vi "AddRequest.vi"(5 "Reply Params Source":refnum<vi>, 7 "Request Params Source":refnum<vi>, 9 "Request Name":string, 10 "Module Name":string="TemplateModule", 11 "Module Ref":refnum<vi>) -> ()   [LabVIEW 2024, in "AddNewEvent.lvlib"]
uses:
  Event/AddNewEvent.lvlib
  <vilib>/Utility/miscctls.llb/LVPositionTypeDef.ctl
  <vilib>/_script/New VI Object TypeDefs/NewVIObject_LVRelativePositionTypeDef.ctl
  <vilib>/_script/New VI Object TypeDefs/NewVIObject_LVRelativeDirectionTypeDef.ctl
  <vilib>/Utility/miscctls.llb/LVPoint32TypeDef.ctl
  <vilib>/event_ctls.llb/lveventtype.ctl
  <vilib>/Utility/traverseref.llb/TRef TravTarget.ctl
  <vilib>/Utility/miscctls.llb/LVPointTypeDef.ctl
  templates/RequestTemplate.vi
  Event/Templates/EHLRequest.vi
  Event/Templates/RequestMessageTemplate.ctl
  <vilib>/addons/analyzer/_analyzerutils.llb/VIAnUtil Check Type If ErrClust.vi
  <vilib>/Utility/traverseref.llb/VI Scripting - Traverse.lvlib
  templates/TemplateModule/TemplateModule.Start.vi
  templates/TemplateModule/TemplateModule.lvclass
  <vilib>/Utility/Data Type/NI_Data Type.lvlib
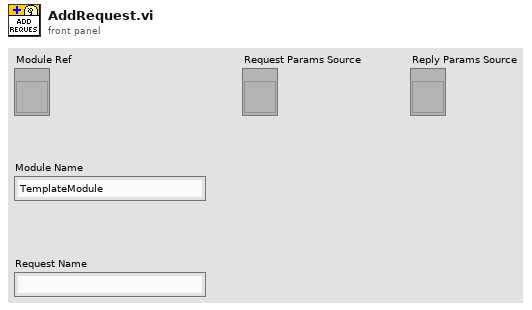
[diagram p1: front panel]
types:
  T1 = typedef "LVPositionTypeDef.ctl" = cluster{"Left":i32, "Top":i32}
  T2 = typedef "lveventtype.ctl" = enum32{"Null", "Timeout", "Annotation Menu Selection", "Annotation Menu Selection?", "App Instance Close", "App Instance Close?", "Autoscale Range Change", "Bookmark Info Change", "Cell Edit", "Cell Edit?", "Cursor Grab", "Cursor Grab?", "Cursor Menu Selection", "Cursor Menu Selection?", "Cursor Move", "Cursor Release", "Data Change", "Direction Change", "Display State Change", "Drag Ended", "Drag Enter", "Drag Leave", "Drag Over", "Drag Source Update", "Drag Starting", "Drag Starting?", "Drop", "Exec State Change", "Key Down", "Key Down?", "Key Repeat", "Key Repeat?", "Key Up", "Listbox Double Click", "Menu Activation?", "Menu Selection (App)", "Menu Selection? (App)", "Menu Selection (User)", "Mouse Down", "Mouse Down?", "Mouse Enter", "Mouse Leave", "Mouse Move", "Mouse Up", "Mouse Wheel", "NI Security User Change (App)", "Pane Size", "Panel Close", "Panel Close?", "Panel Resize", "Plot Attribute Change", "Scale Range Change", "Shortcut Menu Activation?", "Shortcut Menu Selection (App)", "Shortcut Menu Selection? (App)", "Shortcut Menu Selection (User)", "Tree Double Click", "Tree Drag", "Tree Drag?", "Tree Drop", "Tree Drop?", "Tree Item Close", "Tree Item Close?", "Tree Item Open", "Tree Item Open?", "User Event", "Value Change"}
  T3 = cluster{"Event Type":T2, "Reference":refnum<vi>, "Limit (-1=none)":i32, "Lock Panel?":bool}
  T4 = typedef "LVPointTypeDef.ctl" = cluster{"Horizontal":i16, "Vertical":i16}
  T5 = typedef "TRef TravTarget.ctl" = enum16{"FP", "BD", "Other"}
  T6 = enum32{"invalid VI type", "Standard VI", "Control VI", "Global VI", "Polymorphic VI", "Configuration VI", "SubSystem", "Facade VI", "Method VI", "Statechart Diagram VI"}
  T7 = cluster{"Event Type":T2, "Event Registration Index":i32}
  T8 = typedef "NewVIObject_LVRelativePositionTypeDef.ctl" = cluster{"Refnum":refnum<vi>, "Relative Direction":T9, "Point32":T10}
  T9 = typedef "NewVIObject_LVRelativeDirectionTypeDef.ctl" = enum32{"Right", "Left", "Top", "Bottom", "Top Right", "Top Left", "Bottom Right", "Bottom Left"}
  T10 = typedef "LVPoint32TypeDef.ctl" = cluster{"Horizontal":i32, "Vertical":i32}
  T11 = cluster{"Event Type":T2, "Event Registration Index":i32}[]
  T12 = cluster{"Event Type":T2, "Reference":refnum<vi>, "Limit (-1=none)":i32, "Lock Panel?":bool}[]
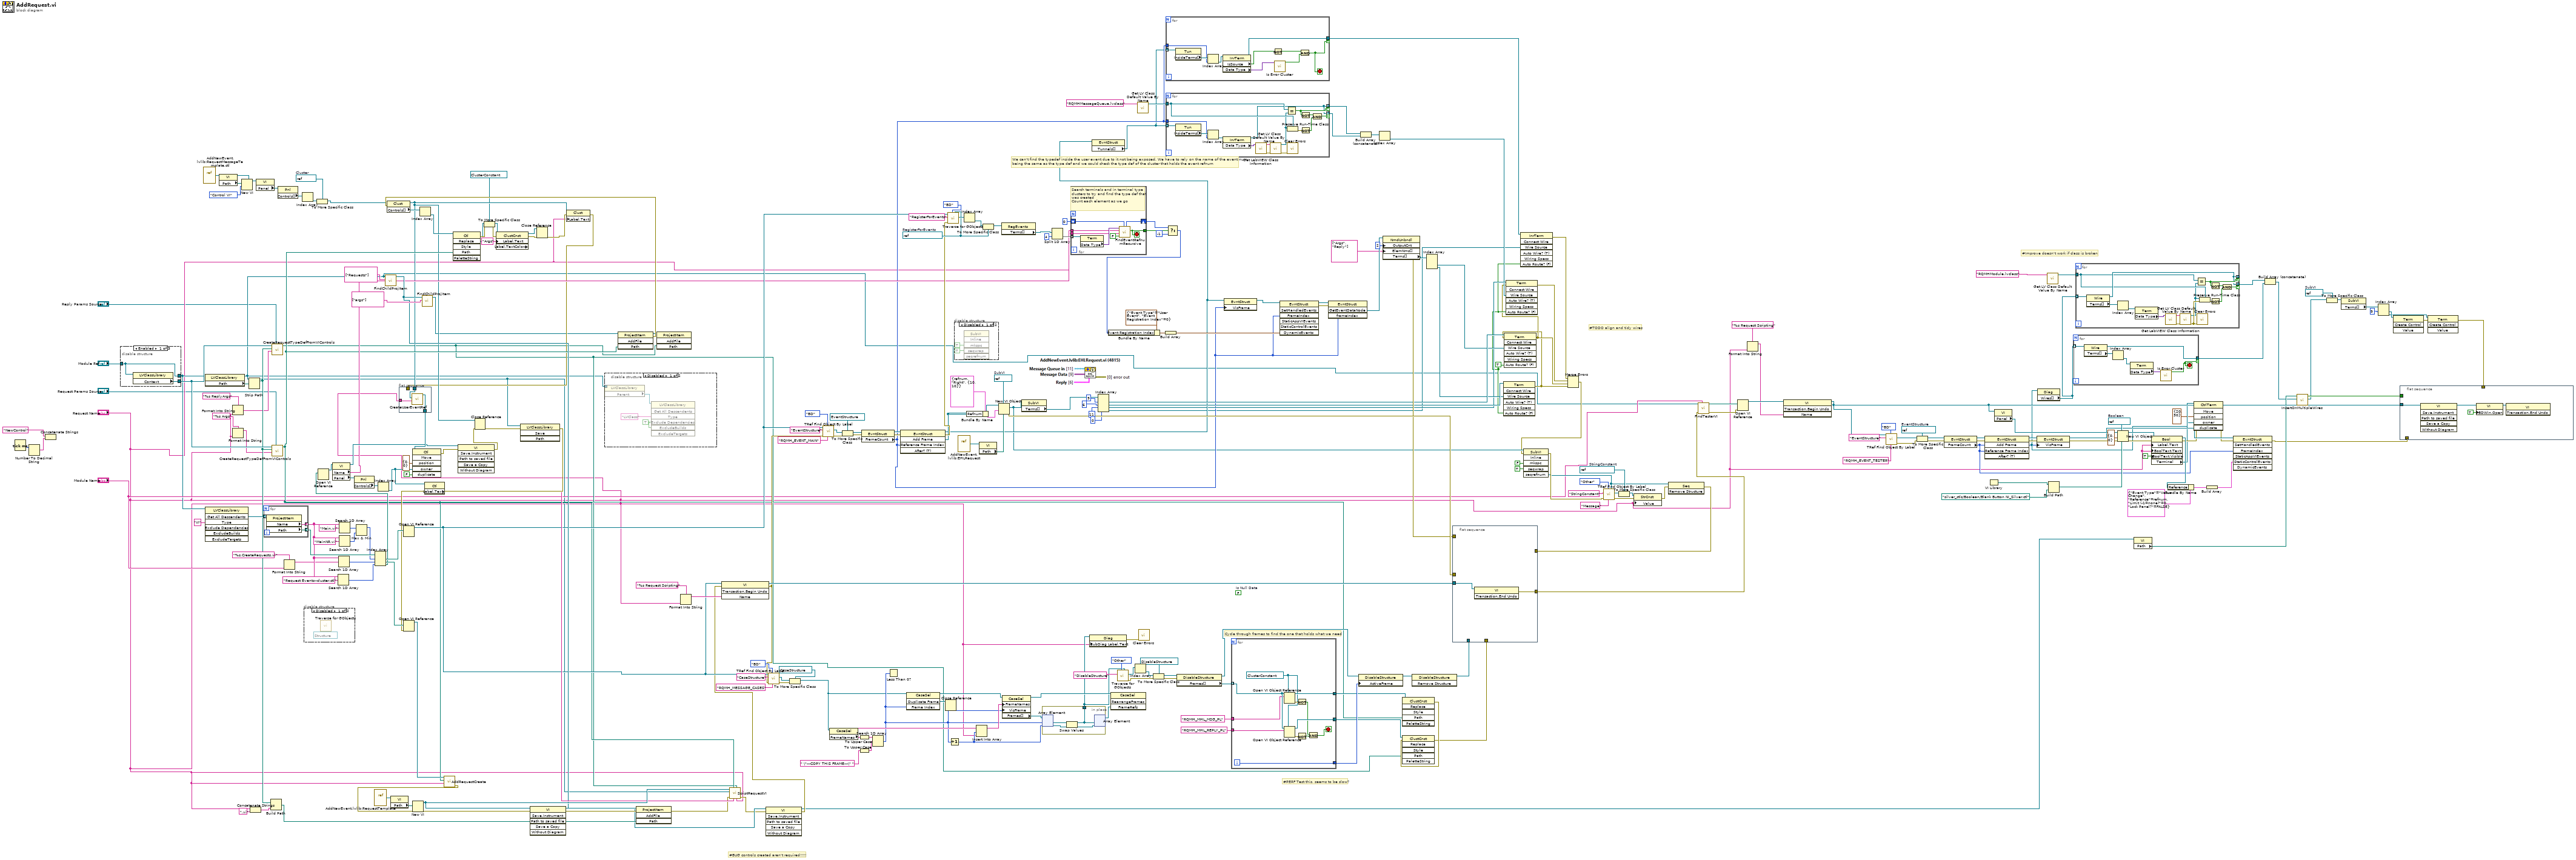
[diagram p0: block diagram]
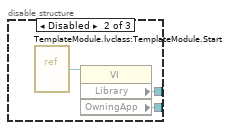
[diagram p2: hidden frame]
diagram:
  w12 = refnum<vi> refnum  # SubVI
  w40 = refnum<vi> refnum  # Boolean
  w58 = refnum<vi> refnum  # EventStructure
  w82 = refnum<vi> refnum  # StringConstant
  w93 = TRUE ("Auto Route? (F)")
  w139 = refnum<vi> refnum  # Cluster
  w170 = refnum<vi> refnum  # RegisterForEvents
  w200 = refnum<vi> refnum  # SubVI
  (unwired) FALSE  # Is Null Data
  # "#BUG controls created aren't required!!!!!"
  # "#Improve doesn't work if class is broken"
  # "#TODO align and tidy wires"
  # "We can't find the typedef inside the user event due to it not being exposed. We have to rely on the name of the event num\nbeing the same as the type def and we could check the type def of the cluster that holds the event refnum"
  # "#PERF Test this, seems to be slow?"
  # "Cycle through frames to find the one that holds what we need"
  n1 = Tick Count (ms)() -> (millisecond timer value=w278:u32)
  n2 = Number To Decimal String(number=w278) -> (decimal integer string=w277:string)  [unwired: 1 in]
  n3 = Concatenate Strings("NewControl", w277) -> ()  [unwired: 1 out]
  n4 = disable-structure shown="Enabled" {
    disable-tunnel: [w282 w285 _] -> w17
    disable-tunnel: [w283 w284 _] -> w213
    disable-tunnel: "Module Ref" -> [w282 _ _]
    frame Enabled {
      n5 = property class="LVClassLibrary"(reference=w282) -> ("Context"=w283:refnum<vi>)  [unwired: 1 in, 2 out]
    }
    frame Disabled {
      n6 = vi-ref "TemplateModule.lvclass:TemplateModule.Start.vi"() -> (w286:refnum<vi>)
      n7 = property class="VI"(reference=w286) -> ("Library"=w285:refnum<vi>, "OwningApp"=w284:refnum<vi>)  [unwired: 1 in, 2 out]
    }
    frame Disabled {
    }
  }
  n8 = vi-ref "AddNewEvent.lvlib:RequestMessageTemplate.ctl"() -> (w147:refnum<vi>)
  n9 = property class="LVClassLibrary"(reference=w17) -> (reference out=w68:refnum<vi>, "Path"=w281:path)  [unwired: 1 in, 1 out]
  n10 = invoke class="LVClassLibrary" method="Get All Descendents"(reference=w17, "Type"="VI") -> ("All Descendents"=w274:refnum<vi>[])  [unwired: 5 in, 6 out]
  n11 = property class="VI"(reference=w147) -> (reference out=w140:refnum<vi>, "Path"=w146:path)  [unwired: 1 in, 1 out]
  n12 = Format Into String(format string="%s ReplyArgs", "Request Name") -> (resulting string=w211:string)  [unwired: 2 in, 1 out]
  n13 = Format Into String(format string="%s Args", "Request Name") -> (resulting string=w208:string)  [unwired: 2 in, 1 out]
  n14 = New VI(5:w140, 9:T6."Control VI" ("vi type (standard vi)"), 10:w146) -> (3:w142:refnum<vi>)  [unwired: 4 in, 1 out]
  n15 = Strip Path(path=w281) -> (stripped path=w212:path)  [unwired: 1 out]
  n16 = Concatenate Strings("Request Name", ".vi" ("string")) -> (w248:string)
  n17 = property class="VI"(reference=w142) -> ("Panel"=w144:refnum<vi>)  [unwired: 1 in, 2 out]
  n18 = for {
    tunnel: w274 -> [w289] mode=indexing
    tunnel: [w288] -> w260 mode=indexing
    tunnel: [w287] -> w269 mode=indexing
    n19 = property class="ProjectItem"(reference=w289) -> ("Name"=w288:string, "Path"=w287:path)  [unwired: 1 in, 2 out]
  }
  n20 = Build Path(base path=w212, name or relative path=w248) -> (appended path=w247:path)
  n21 = call "CreateRequestTypeDefFromVIControls.vi"("VI Refnum"="Reply Params Source", "Control Name"=w211, "SaveFolderPath"=w212, "Application in"=w213) -> ("TypeDef Path"=w70:path)  [unwired: 6 in, 1 out]
  n22 = call "CreateRequestTypeDefFromVIControls.vi"("VI Refnum"="Request Params Source", "Control Name"=w208, "SaveFolderPath"=w212, "Application in"=w213) -> ("TypeDef Path"=w135:path)  [unwired: 6 in, 1 out]
  n23 = property class="Pnl"(reference=w144) -> ("Controls[]"=w143:refnum<vi>[])  [unwired: 1 in, 2 out]
  n24 = Format Into String(format string="%s.CreateRequests.vi" ("element"), "Module Name") -> (resulting string=w239:string)  [unwired: 2 in, 1 out]
  n25 = Index Array(array=w143) -> (element=w141:refnum<vi>)  [unwired: 1 in]
  n26 = disable-structure shown="Disabled" {
    frame Disabled {
      (unwired) refnum<vi> refnum ("Struct Refnum")
      n27 = call <vilib>:"Traverse for GObjects.vi"() -> ()  [unwired: 8 in, 4 out]
    }
    frame Enabled {
    }
  }
  n28 = To More Specific Class(target class=w139, reference=w141) -> (specific class reference=w138:refnum<vi>)  [unwired: 1 in, 1 out]
  n29 = Search 1D Array(1D array=w260, element="Request Events--cluster.ctl") -> (index of element=w259:i32)  [unwired: 1 in]
  n30 = Search 1D Array(1D array=w260, element=w239) -> (index of element=w268:i32)  [unwired: 1 in]
  n31 = Search 1D Array(1D array=w260, element="Main.vi") -> (index of element=w271:i32)  [unwired: 1 in]
  n32 = Search 1D Array(1D array=w260, element="MainNR.vi") -> (index of element=w270:i32)  [unwired: 1 in]
  n33 = Max & Min(x=w271, y=w270) -> (max(x,y)=w267:i32)  [unwired: 1 out]
  n34 = vi-ref "AddNewEvent.lvlib:RequestTemplate.vi"() -> (w280:refnum<vi>)
  n35 = Index Array(array=w269, index #1=w267, index #2=w268, index #3=w259) -> (element #1=w265:path, element #2=w266:path, element #3=w255:path)
  n36 = Open VI Reference(vi path=w255) -> (vi reference=w256:refnum<vi>)  [unwired: 5 in, 1 out]
  n37 = property class="VI"(reference=w256) -> (reference out=w205:refnum<vi>, "Name"=w157:string, "Panel"=w258:refnum<vi>)  [unwired: 1 in, 1 out]
  n38 = property class="Pnl"(reference=w258) -> ("Controls[]"=w257:refnum<vi>[])  [unwired: 1 in, 2 out]
  n39 = Index Array(array=w257) -> (element=w245:refnum<vi>)  [unwired: 1 in]
  n40 = call "FindChildProjItem.vi"("Level"=string[] ["Requests"], "ProjectItem in"=w68) -> ("Found or Orig"=w201:refnum<vi>)  [unwired: 8 in, 1 out]
  n41 = property class="VI"(reference=w280) -> ("Path"=w279:path)  [unwired: 1 in, 2 out]
  n42 = flat-sequence {
    tunnel: [w292] -> w252
    tunnel: "Request Name" -> [w291]
    tunnel: w131 -> [w290]
    tunnel: w129 -> [_]
    frame #0 {
      n43 = call "CreateUserEventRef.vi"("Label.Text"=w291, "referenceToEventRef"=w290) -> ("UserEventCtlRef"=w292:refnum<vi>)  [unwired: 9 in]
    }
  }
  n44 = Open VI Reference(vi path=w265) -> (vi reference=w160:refnum<vi>)  [unwired: 5 in, 1 out]
  n45 = invoke class="Ctl" method="Move"(reference=w252, "position"=T1 {"Left"=0, "Top"=0}, "owner"=w245, "duplicate"=FALSE ("Duplicate? (F)")) -> (error out=w207:errorcluster)  [unwired: 2 in, 5 out]
  n46 = call "FindChildProjItem.vi"("Level"=string[] ["args"], "ProjectItem in"=w201) -> ("Found or Orig"=w120:refnum<vi>)  [unwired: 8 in, 1 out]
  n47 = property class="Ctl"(reference=w245) -> ("Label.Text"=w244:string)  [unwired: 1 in, 2 out]
  n48 = invoke class="VI" method="Save.Instrument"(reference=w205, error in=w207) -> (error out=w206:errorcluster)  [unwired: 4 in, 5 out]
  n49 = disable-structure shown="Disabled" {
    disable-tunnel: w68 -> [w296 _]
    frame Disabled {
      w294 = TRUE ("ExcludeDependencies")
      n50 = property class="LVClassLibrary"(reference=w296) -> ("Parent"=w295:refnum<vi>)  [unwired: 1 in, 2 out]
      n51 = invoke class="LVClassLibrary" method="Get All Descendents"(reference=w295, "Type"="LVClass", "Exclude Dependencies"=w294, "ExcludeBuilds"=w294) -> ()  [unwired: 3 in, 7 out]
    }
    frame Enabled {
    }
  }
  n52 = invoke class="ProjectItem" method="AddFile"(reference=w120, "Path"=w135) -> (reference out=w121:refnum<vi>, error out=w204:errorcluster)  [unwired: 2 in, 2 out]
  n53 = property class="Clust"(reference=w138, error in=w204) -> (reference out=w131:refnum<vi>, "Controls[]"=w137:refnum<vi>[])  [unwired: 1 out]
  n54 = Index Array(array=w137) -> (element=w136:refnum<vi>)  [unwired: 1 in]
  n55 = invoke class="Ctl" method="Replace"(reference=w136, "Path"=w135) -> (error out=w128:errorcluster, "Replace"=w126:refnum<vi>)  [unwired: 4 in, 4 out]
  n56 = Close Reference(reference=w131, error in (no error)=w206) -> (error out=w263:errorcluster)
  n57 = To More Specific Class(target class=refnum<vi> refnum ("ClustCnst Refnum"), reference=w126, error in=w128) -> (specific class reference=w124:refnum<vi>, error out=w127:errorcluster)
  n58 = property class="ClustCnst" props=["Label", "Text", "Label", "TextColors"](reference=w124, error in=w127, "Label.Text"="Args") -> (reference out=w133:refnum<vi>, error out=w132:errorcluster)  [unwired: 1 out]
  n59 = invoke class="LVClassLibrary" method="Save"(reference=w68, error in=w263) -> (error out=w254:errorcluster)  [unwired: 2 in, 3 out]
  n60 = Open VI Reference(vi path=w266, error in (no error)=w254) -> (vi reference=w264:refnum<vi>)  [unwired: 4 in, 1 out]
  n61 = call "AddRequestCreate.vi"("New Name"="Request Name", "TypeDefPath"=w135, "VI in"=w264) -> ("error out"=w149:errorcluster)  [unwired: 8 in]
  n62 = New VI(8:w149, 10:w279) -> (0:w251:errorcluster, 3:w246:refnum<vi>)  [unwired: 5 in]
  n63 = invoke class="VI" method="Save.Instrument"(reference=w246, error in=w251, "Path to saved file"=w247) -> (reference out=w48:refnum<vi>, error out=w250:errorcluster)  [unwired: 3 in, 4 out]
  n64 = Close Reference(reference=w133, error in (no error)=w132) -> (error out=w130:errorcluster)
  n65 = property class="Clust"(reference=w131, error in=w130, "Label.Text"="Request Name") -> (error out=w129:errorcluster)  [unwired: 1 out]
  n66 = invoke class="ProjectItem" method="AddFile"(reference=w201, error in=w250, "Path"=w247) -> (error out=w148:errorcluster)  [unwired: 1 in, 3 out]
  n67 = invoke class="ProjectItem" method="AddFile"(reference=w121, "Path"=w70) -> ()  [unwired: 2 in, 4 out]
  n68 = Format Into String(format string="%s Request Scripting", "Request Name") -> (resulting string=w178:string)  [unwired: 2 in, 1 out]
  n69 = call "ScriptRequestVI.vi"("Request Name"="Request Name", "REPLYTypeDef Path"=w70, "EventClusterName"=w244, "REQTypeDef Path"=w135, "error in (no error)"=w148, "Module Ref"=w68, "VI in"=w246) -> ("error out"=w47:errorcluster)  [unwired: 4 in]
  n70 = invoke class="VI" method="Save.Instrument"(reference=w48, error in=w47) -> (reference out=w45:refnum<vi>, error out=w46:errorcluster)  [unwired: 4 in, 4 out]
  n71 = invoke class="VI" method="Transaction.Begin Undo"(reference=w160, error in=w46, "Name"=w178) -> (reference out=w177:refnum<vi>, error out=w159:errorcluster)  [unwired: 1 in, 2 out]
  n72 = call <vilib>:"TRef Find Object By Label.vi"("Label"="RQMH_MESSAGE_CASES", "Traverse Target"=TRef_TravTarget."BD", "error in (no error)"=w159, "Class Name"="CaseStructure", "VI Ref"=w160) -> ("error out"=w181:errorcluster, "Found Obj Ref"=w182:refnum<vi>)  [unwired: 3 in, 2 out]
  n73 = To More Specific Class(target class=refnum<vi> refnum ("CaseSel Refnum"), reference=w182, error in=w181) -> (specific class reference=w180:refnum<vi>)  [unwired: 1 out]
  n74 = call <vilib>:"TRef Find Object By Label.vi"("Label"="RQMH_EVENT_MAIN", "Traverse Target"=TRef_TravTarget."BD", "error in (no error)"=w159, "Class Name"="EventStructure", "VI Ref"=w160) -> ("error out"=w196:errorcluster, "Found Obj Ref"=w195:refnum<vi>)  [unwired: 3 in, 2 out]
  n75 = property class="CaseSel"(reference=w180) -> ("FrameNames"=w225:string[])  [unwired: 1 in, 2 out]
  n76 = To More Specific Class(target class=refnum<vi> refnum ("EvntStruct Refnum"), reference=w195, error in=w196) -> (specific class reference=w191:refnum<vi>, error out=w193:errorcluster)
  n77 = To Upper Case(1:" \"---COPY THIS FRAME---\" " ("key")) -> (0:w237:string)
  n78 = To Upper Case(1:w225) -> (0:w238:string[])
  n79 = property class="EvntStruct"(reference=w191, error in=w193) -> (reference out=w174:refnum<vi>, error out=w192:errorcluster, "FrameCount"=w97:i32)
  n80 = Search 1D Array(1D array=w238, element=w237) -> (index of element=w222:i32)  [unwired: 1 in]
  n81 = Less Than 0?(x=w222) -> ()  [unwired: 1 out]
  n82 = invoke class="EvntStruct" method="Add Frame"(reference=w174, error in=w192, "Reference Frame Index"=w97) -> (reference out=w107:refnum<vi>, error out=w158:errorcluster, "Add Frame"=w108:refnum<vi>)  [unwired: 2 in, 2 out]
  n83 = invoke class="CaseSel" method="Duplicate Frame"(reference=w180, "Frame Index"=w222) -> (reference out=w235:refnum<vi>, "Duplicate Frame"=w231:refnum<vi>)  [unwired: 2 in, 2 out]
  n84 = Close Reference(reference=w231) -> ()  [unwired: 1 in, 1 out]
  n85 = call <vilib>:"Traverse for GObjects.vi"("Other Refnum"=w170, "Traverse Target"=TRef_TravTarget."BD", "error in (no error)"=w158, "Class Name"="RegisterForEvents", "VI Refnum"=w160) -> ("References"=w171:refnum<vi>[])  [unwired: 3 in, 3 out]
  n86 = Increment(x=w222) -> (x+1=w223:i32)
  n87 = disable-structure shown="Disabled" {
    frame Disabled {
      n88 = invoke class="SubVI" method="Inline"("mkspc"=TRUE ("Make Space in Block Diagram"), "seqwrap"=TRUE ("Wrap in Sequence")) -> ()  [unwired: 4 in, 6 out]
    }
    frame Enabled {
    }
  }
  n89 = vi-ref "AddNewEvent.lvlib:EHLRequest.vi"() -> (w189:refnum<vi>)
  n90 = Index Array(array=w171) -> (element=w169:refnum<vi>)  [unwired: 1 in]
  n91 = Bundle By Name(cluster=T8 {"Refnum"=refnum, "Relative Direction"=enum."Right", "Point32"={"Horizontal"=10, "Vertical"=10}} ("Relative Position"), "Refnum"=w108) -> (w187:T8)
  n92 = Insert Into Array(array=w225, index=w223, new element="Request Name") -> (w224:string[])
  n93 = property class="VI"(reference=w189) -> ("Path"=w188:path)  [unwired: 1 in, 2 out]
  n94 = To More Specific Class(target class=w170, reference=w169) -> (specific class reference=w168:refnum<vi>)  [unwired: 1 in, 1 out]
  n95 = New VI Object(vi object class=w200, owner refnum=w108, position/next to=w187, 6:w188) -> (object refnum=w89:refnum<vi>, 0:w175:errorcluster)  [unwired: 4 in]
  n96 = property class="RegEvents"(reference=w168) -> ("Terms[]"=w167:refnum<vi>[])  [unwired: 1 in, 2 out]
  n97 = property class="CaseSel"(reference=w235, "FrameNames"=w224, "VisFrame"=w222) -> (reference out=w234:refnum<vi>, "Frames[]"=w233:refnum<vi>[])  [unwired: 1 in, 1 out]
  n98 = property class="SubVI"(reference=w89) -> ("Terms[]"=w116:refnum<vi>[])  [unwired: 1 in, 2 out]
  n99 = in-place {
    in-place-border: [w299] -> w226
    n100 = in-place-array #1(w233, w222, w223) -> (w302:refnum<vi>, w301:refnum<vi>)
    n101 = Swap Values(12:w302, 14:w301) -> (1:w299:refnum<vi>, 3:w300:refnum<vi>)  [unwired: 1 in]
    n102 = in-place-array #1(w299, w300) -> (w232:refnum<vi>[])  [unwired: 2 out]
  }
  n103 = Split 1D Array(array=w167, index=4) -> (second subarray=w165:refnum<vi>[])  [unwired: 1 out]
  n104 = for {
    tunnel: w165 -> [w310] mode=indexing
    tunnel: "Request Name" -> [w305]
    shift-right: [w309] -> w161
    shift-left: 0 -> [w308]
    tunnel: [w307] -> w163
    tunnel: w157 -> [w304]
    stop <- w307 stop-if-true
    # "Search terminals and in terminal type clusters to try and find the type def that was created\nCount each element as we go"
    n105 = property class="Term"(reference=w310) -> ("Data Type"=w306:variant)  [unwired: 1 in, 2 out]
    n106 = call "FindEventRefnumRecursive.vi"("count in"=w308, "InNamedTypedef?"=FALSE, "Event name"=w305, "Event holder typedef"=w304, "Data Type"=w306) -> ("Found?"=w307:bool, "count out"=w309:i32)  [unwired: 5 in]
  }
  n107 = property class="Diag"(reference=w226, "SubDiag Label.Text"="Request Name") -> (error out=w230:errorcluster)  [unwired: 1 in, 1 out]
  n108 = property class="EvntStruct"(reference=w107) -> ("Tunnels[]"=w96:refnum<vi>[])  [unwired: 1 in, 2 out]
  n109 = Index Array(array=w116, index #1=9 ("index"), index #2=6 ("index"), index #3=11 ("index"), index #4=0 ("index")) -> (element #1=w112:refnum<vi>, element #2=w111:refnum<vi>, element #3=w101:refnum<vi>, element #4=w94:refnum<vi>)
  n110 = invoke class="CaseSel" method="RearrangeFrames"(reference=w234, "FrameRefs"=w232) -> ()  [unwired: 2 in, 4 out]
  n111 = call <vilib>:"Traverse for GObjects.vi"("Other Refnum"=w226, "Traverse Target"=TRef_TravTarget."Other", "Class Name"="DisableStructure") -> ("error out"=w229:errorcluster, "References"=w228:refnum<vi>[])  [unwired: 5 in, 2 out]
  n112 = Index Array(array=w228) -> (element=w227:refnum<vi>)  [unwired: 1 in]
  n113 = call <vilib>:"Get LV Class Default Value By Name.vi"("class name"="RQMHMessageQueue.lvclass") -> ("object"=w105:refnum<class>)  [unwired: 9 in, 1 out]
  n114 = call <vilib>:"Clear Errors.vi"("error in (no error)"=w230) -> ()  [unwired: 5 in, 2 out]
  n115 = To More Specific Class(target class=refnum<vi> refnum ("DisableStructure Refnum"), reference=w227, error in=w229) -> (specific class reference=w221:refnum<vi>, error out=w220:errorcluster)
  n116 = for {
    tunnel: w96 -> [w320] mode=indexing
    tunnel: w97 -> [w317]
    tunnel: [w311] -> w95 if=w312
    stop <- w312 stop-if-true
    n117 = property class="Tun"(reference=w320) -> ("InsideTerms[]"=w319:refnum<vi>[])  [unwired: 1 in, 2 out]
    n118 = Index Array(array=w319, index=w317) -> (element=w318:refnum<vi>)
    n119 = property class="InrTerm"(reference=w318) -> (reference out=w311:refnum<vi>, "IsSource"=w314:bool, "Data Type"=w316:variant)  [unwired: 1 in, 1 out]
    n120 = Not(x=w314) -> (.not. x?=w313:bool)
    n121 = call <vilib>:"Is Error Cluster.vi"("variant"=w316) -> ("is error cluster?"=w315:bool)  [unwired: 9 in, 1 out]
    n122 = And(x=w313, y=w315) -> (x .and. y?=w312:bool)
  }
  n123 = for {
    tunnel: w96 -> [w336] mode=indexing
    tunnel: w105 -> [w330]
    tunnel: [w321] -> w104 mode=indexing if=w328
    tunnel: [w321] -> w103 mode=indexing if=w325
    tunnel: w97 -> [w324]
    n124 = property class="Tun"(reference=w336) -> ("InsideTerms[]"=w335:refnum<vi>[])  [unwired: 1 in, 2 out]
    n125 = Index Array(array=w335, index=w324) -> (element=w334:refnum<vi>)
    n126 = property class="InrTerm"(reference=w334) -> (reference out=w321:refnum<vi>, "Data Type"=w333:variant)  [unwired: 1 in, 1 out]
    n127 = call <vilib>:"Get LabVIEW Class Information.vi"("variant"=w333) -> ("error out"=w323:errorcluster, "LabVIEW class file name"=w332:string)  [unwired: 8 in, 1 out]
    n128 = call <vilib>:"Get LV Class Default Value By Name.vi"("error in (no error)"=w323, "class name"=w332) -> ("error out"=w322:errorcluster, "object"=w329:refnum<class>)  [unwired: 8 in]
    n129 = Equal?(x=w330, y=w329) -> (x = y?=w328:bool)
    n130 = Preserve Run-Time Class(object in=w329, 2:w330) -> (error out=w331:errorcluster)  [unwired: 1 in, 1 out]
    n131 = call <vilib>:"Clear Errors.vi"("error in (no error)"=w322) -> ()  [unwired: 5 in, 2 out]
    n132 = Not(x=w328) -> (.not. x?=w326:bool)
    n133 = Not(x=w331) -> (.not. x?=w327:bool)
    n134 = And(x=w326, y=w327) -> (x .and. y?=w325:bool)
  }
  n135 = Select(t=w161, s=w163, f=-1) -> (s? t:f=w150:i32)
  n136 = Bundle By Name(cluster=T7 {"Event Type"=enum."User Event", "Event Registration Index"=0} ("Dynamic Events"), "Event Registration Index"=w150) -> (w156:T7)
  n137 = Build Array(w156) -> (w154:T11)
  n138 = property class="DisableStructure"(reference=w221, error in=w220) -> (reference out=w216:refnum<vi>, "Frames[]"=w219:refnum<vi>[])  [unwired: 1 out]
  n139 = property class="EvntStruct"(reference=w107, "VisFrame"=w97) -> (reference out=w123:refnum<vi>)  [unwired: 1 in, 1 out]
  n140 = for {
    tunnel: w219 -> [w348] mode=indexing
    tunnel: "RQMH_MHL_REPLY_PL" -> [w346]
    tunnel: "RQMH_MHL_MSG_PL" -> [w345]
    tunnel: [w344] -> w214
    tunnel: [w343] -> w73
    tunnel: [w341] -> w215
    i -> [w341]
    stop <- w337 stop-if-true
    w342 = refnum<vi> refnum ("ClustCnst Refnum")
    n141 = Open VI Object Reference(7:w342, 10:w345, 11:w348) -> (0:w347:errorcluster, 3:w344:refnum<vi>)  [unwired: 1 in]
    n142 = Open VI Object Reference(7:w342, 10:w346, 11:w348) -> (0:w340:errorcluster, 3:w343:refnum<vi>)  [unwired: 1 in]
    n143 = Not(x=w347) -> (.not. x?=w338:bool)
    n144 = Not(x=w340) -> (.not. x?=w339:bool)
    n145 = And(x=w338, y=w339) -> (x .and. y?=w337:bool)
  }
  n146 = invoke class="EvntStruct" method="SetHandledEvents"(reference=w123, "FrameIndex"=w97, "DynamicEvents"=w154) -> (reference out=w152:refnum<vi>, error out=w153:errorcluster)  [unwired: 4 in, 5 out]
  n147 = invoke class="EvntStruct" method="GetEventDataNode"(reference=w152, error in=w153, "frameIndex"=w97) -> ("GetEventDataNode"=w151:refnum<vi>)  [unwired: 1 in, 3 out]
  n148 = property class="DisableStructure"(reference=w216, "ActiveFrame"=w215) -> (reference out=w176:refnum<vi>)  [unwired: 1 in, 1 out]
  n149 = Build Array (concatenate)(w104, w103) -> (w102:refnum<vi>[])
  n150 = Index Array(array=w102) -> (element=w100:refnum<vi>)  [unwired: 1 in]
  n151 = property class="NmdUnbndl"(reference=w151, "OutputCnt"=2 ("Output Count"), "ElemNms[]"=string[] ["Args", "Reply"] ("Element Names[]")) -> (error out=w122:errorcluster, "Terms[]"=w117:refnum<vi>[])  [unwired: 1 in, 1 out]
  n152 = invoke class="ClustCnst" method="Replace"(reference=w214, "Path"=w135) -> (error out=w72:errorcluster)  [unwired: 4 in, 5 out]
  n153 = invoke class="ClustCnst" method="Replace"(reference=w73, error in=w72, "Path"=w70) -> (error out=w71:errorcluster)  [unwired: 3 in, 5 out]
  n154 = invoke class="DisableStructure" method="Remove Structure"(reference=w176) -> (reference out=w74:refnum<vi>)  [unwired: 2 in, 2 out]
  n155 = Index Array(array=w117) -> (element #2=w110:refnum<vi>, element #3=w109:refnum<vi>)  [unwired: 3 in, 1 out]
  n156 = flat-sequence {
    tunnel: w177 -> [w350]
    tunnel: w74 -> [_]
    tunnel: w175 -> [_]
    tunnel: w122 -> [_]
    tunnel: w75 -> [_]
    tunnel: w71 -> [_]
    tunnel: [w349] -> w65
    frame #0 {
      n157 = invoke class="VI" method="Transaction.End Undo"(reference=w350) -> (error out=w349:errorcluster)  [unwired: 2 in, 2 out]
    }
  }
  n158 = invoke class="Term" method="Connect Wire"(reference=w111, "Wire Source"=w109, "Auto Route? (F)"=w93) -> (error out=w90:errorcluster)  [unwired: 4 in, 6 out]
  n159 = invoke class="Term" method="Connect Wire"(reference=w112, error in=w90, "Wire Source"=w110, "Auto Route? (F)"=w93) -> (error out=w91:errorcluster)  [unwired: 3 in, 6 out]
  n160 = invoke class="Term" method="Connect Wire"(reference=w101, error in=w91, "Wire Source"=w100, "Auto Route? (F)"=w93) -> (error out=w99:errorcluster)  [unwired: 3 in, 6 out]
  n161 = invoke class="InrTerm" method="Connect Wire"(reference=w95, "Wire Source"=w94, "Auto Route? (F)"=w93) -> (error out=w92:errorcluster)  [unwired: 4 in, 6 out]
  n162 = Merge Errors(w92, w99, w91, w90) -> (w87:errorcluster)
  n163 = invoke class="SubVI" method="Inline"(reference=w89, error in=w87, "mkspc"=FALSE ("Make Space in Block Diagram"), "seqwrap"=TRUE ("Wrap in Sequence")) -> (error out=w79:errorcluster, "seqrefnum"=w77:refnum<vi>)  [unwired: 2 in, 4 out]
  n164 = call <vilib>:"TRef Find Object By Label.vi"("Other Refnum"=w77, "Label"="Message" ("name/order"), "Traverse Target"=TRef_TravTarget."Other", "error in (no error)"=w79, "Class Name"="StringConstant") -> ("error out"=w78:errorcluster, "Found Obj Ref"=w81:refnum<vi>)  [unwired: 3 in, 2 out]
  n165 = To More Specific Class(target class=w82, reference=w81) -> (specific class reference=w80:refnum<vi>)  [unwired: 1 in, 1 out]
  n166 = property class="StrCnst"(reference=w80, error in=w78, "Value"="Request Name") -> (error out=w76:errorcluster)  [unwired: 1 out]
  n167 = invoke class="Seq" method="Remove Structure"(reference=w77, error in=w76) -> (error out=w75:errorcluster)  [unwired: 1 in, 2 out]
  n168 = call "FindTesterVI.vi"("Module Name"="Module Name", "error in (no error)"=w65, "module ref"=w68) -> ("error out"=w66:errorcluster, "TesterPath"=w67:path)  [unwired: 7 in]
  n169 = Open VI Reference(vi path=w67, error in (no error)=w66) -> (vi reference=w64:refnum<vi>)  [unwired: 4 in, 1 out]
  n170 = Format Into String(format string="%s Request Scripting" ("Name"), "Request Name") -> (resulting string=w59:string)  [unwired: 2 in, 1 out]
  n171 = invoke class="VI" method="Transaction.Begin Undo"(reference=w64, "Name"=w59) -> (reference out=w39:refnum<vi>)  [unwired: 2 in, 3 out]
  n172 = call <vilib>:"TRef Find Object By Label.vi"("Label"="RQMH_EVENT_TESTER", "Traverse Target"=TRef_TravTarget."BD", "Class Name"="EventStructure", "VI Ref"=w39) -> ("error out"=w52:errorcluster, "Found Obj Ref"=w56:refnum<vi>)  [unwired: 4 in, 2 out]
  n173 = To More Specific Class(target class=w58, reference=w56, error in=w52) -> (specific class reference=w57:refnum<vi>, error out=w53:errorcluster)
  n174 = property class="EvntStruct"(reference=w57, error in=w53) -> (reference out=w55:refnum<vi>, error out=w54:errorcluster, "FrameCount"=w21:i32)
  n175 = invoke class="EvntStruct" method="Add Frame"(reference=w55, error in=w54, "Reference Frame Index"=w21) -> (reference out=w51:refnum<vi>, error out=w50:errorcluster, "Add Frame"=w16:refnum<vi>)  [unwired: 2 in, 2 out]
  n176 = VI Library() -> (path=w43:path)
  n177 = property class="VI"(reference=w39) -> ("Panel"=w38:refnum<vi>)  [unwired: 1 in, 2 out]
  n178 = property class="EvntStruct"(reference=w51, error in=w50, "VisFrame"=w21) -> (reference out=w34:refnum<vi>, error out=w44:errorcluster)
  n179 = property class="Diag"(reference=w16) -> ("Wires[]"=w20:refnum<vi>[])  [unwired: 1 in, 2 out]
  n180 = call <vilib>:"Get LV Class Default Value By Name.vi"("class name"="RQMHModule.lvclass") -> ("object"=w23:refnum<class>)  [unwired: 9 in, 1 out]
  n181 = Build Path(base path=w43, name or relative path=path "silver_ctls/Boolean/Blank Button NI_Silver.ctl") -> (appended path=w41:path)
  n182 = for {
    tunnel: w20 -> [w356] mode=indexing
    tunnel: [w352] -> w49 if=w351
    stop <- w351 stop-if-true
    n183 = property class="Wire"(reference=w356) -> (reference out=w352:refnum<vi>, "Terms[]"=w355:refnum<vi>[])  [unwired: 1 in, 1 out]
    n184 = Index Array(array=w355) -> (element=w354:refnum<vi>)  [unwired: 1 in]
    n185 = property class="Term"(reference=w354) -> ("Data Type"=w353:variant)  [unwired: 1 in, 2 out]
    n186 = call <vilib>:"Is Error Cluster.vi"("variant"=w353) -> ("is error cluster?"=w351:bool)  [unwired: 9 in, 1 out]
  }
  n187 = for {
    tunnel: w20 -> [w371] mode=indexing
    tunnel: w23 -> [w358]
    tunnel: [w361] -> _ mode=indexing if=w366
    tunnel: [w361] -> w19 mode=indexing if=w363
    n188 = property class="Wire"(reference=w371) -> (reference out=w361:refnum<vi>, "Terms[]"=w370:refnum<vi>[])  [unwired: 1 in, 1 out]
    n189 = Index Array(array=w370) -> (element=w369:refnum<vi>)  [unwired: 1 in]
    n190 = property class="Term"(reference=w369) -> ("Data Type"=w360:variant)  [unwired: 1 in, 2 out]
    n191 = call <vilib>:"Get LabVIEW Class Information.vi"("variant"=w360) -> ("error out"=w362:errorcluster, "LabVIEW class file name"=w368:string)  [unwired: 8 in, 1 out]
    n192 = call <vilib>:"Get LV Class Default Value By Name.vi"("error in (no error)"=w362, "class name"=w368) -> ("error out"=w359:errorcluster, "object"=w357:refnum<class>)  [unwired: 8 in]
    n193 = Equal?(x=w358, y=w357) -> (x = y?=w366:bool)
    n194 = call <vilib>:"Clear Errors.vi"("error in (no error)"=w359) -> ()  [unwired: 5 in, 2 out]
    n195 = Preserve Run-Time Class(object in=w357, error in=w359, 2:w358) -> (error out=w367:errorcluster)  [unwired: 1 out]
    n196 = Not(x=w366) -> (.not. x?=w364:bool)
    n197 = Not(x=w367) -> (.not. x?=w365:bool)
    n198 = And(x=w364, y=w365) -> (x .and. y?=w363:bool)
  }
  n199 = New VI Object(vi object class=w40, owner refnum=w38, position/next to=T4 {"Horizontal"=0, "Vertical"=0} ("location"), 6:w41, 8:w44) -> (object refnum=w36:refnum<vi>, 0:w35:errorcluster)  [unwired: 3 in]
  n200 = property class="VI"(reference=w45) -> ("Path"=w22:path)  [unwired: 1 in, 2 out]
  n201 = property class="Bool"(reference=w36, error in=w35, "Label.Text"="Request Name", "BoolText.Text"="Request Name", "BoolText.Visible"=TRUE ("Boolean Text.Visible")) -> (reference out=w30:refnum<vi>, error out=w28:errorcluster, "Terminal"=w26:refnum<vi>)
  n202 = Bundle By Name(cluster=T3 {"Event Type"=enum."Value Change", "Reference"=refnum, "Limit (-1=none)"=0, "Lock Panel?"=FALSE} ("Static Control Events"), "Reference"=w30) -> (w32:T3)
  n203 = invoke class="CtrlTerm" method="Move"(reference=w26, error in=w28, "position"=T1 {"Left"=20, "Top"=30}, "owner"=w16) -> (error out=w27:errorcluster)  [unwired: 2 in, 5 out]
  n204 = Build Array(w32) -> (w31:T12)
  n205 = invoke class="EvntStruct" method="SetHandledEvents"(reference=w34, error in=w27, "FrameIndex"=w21, "StaticControlEvents"=w31) -> (error out=w15:errorcluster)  [unwired: 3 in, 6 out]
  n206 = Build Array (concatenate)(w19, w49) -> (w18:refnum<vi>[])
  n207 = call "InsertOnMultipleWires.vi"("Wire Array"=w18, "To Insert"=w22) -> ("Inserted"=w13:refnum<vi>, "Done?"=w14:bool)  [unwired: 8 in]
  n208 = To More Specific Class(target class=w12, reference=w13) -> (specific class reference=w11:refnum<vi>)  [unwired: 1 in, 1 out]
  n209 = property class="SubVI"(reference=w11) -> ("Terms[]"=w10:refnum<vi>[])  [unwired: 1 in, 2 out]
  n210 = Index Array(array=w10, index #1=9 ("index")) -> (element #1=w8:refnum<vi>, element #2=w7:refnum<vi>)  [unwired: 1 in]
  n211 = invoke class="Term" method="Create Control"(reference=w8) -> (error out=w6:errorcluster)  [unwired: 3 in, 3 out]
  n212 = flat-sequence {
    tunnel: w39 -> [w372]
    tunnel: w15 -> [_]
    tunnel: w14 -> [_]
    tunnel: w5 -> [_]
    frame #0 {
      n213 = invoke class="VI" method="Save.Instrument"(reference=w372) -> (reference out=w373:refnum<vi>)  [unwired: 5 in, 5 out]
      n214 = property class="VI"(reference=w373, "BDWin.Open"=TRUE ("Block Diagram Window:Open")) -> (reference out=w375:refnum<vi>)  [unwired: 1 in, 1 out]
      n215 = invoke class="VI" method="Transaction.End Undo"(reference=w375) -> ()  [unwired: 2 in, 3 out]
    }
  }
  n216 = invoke class="Term" method="Create Control"(reference=w7, error in=w6) -> (error out=w5:errorcluster)  [unwired: 2 in, 3 out]
